vi "Approach_runningAverage_VUW.vi"(7 "Computer called (T/F)":bool) -> ()   [LabVIEW 2023]
uses:
  Sub_Vi/TypeDefsControls/Zposition.ctl
  Sub_Vi/TypeDefsControls/Piezo Velocity.ctl
  Sub_Vi/TypeDefsControls/Voltage.ctl
  Sub_Vi/TypeDefsControls/Xposition.ctl
  Sub_Vi/TypeDefsControls/Yposition.ctl
  Sub_Vi/TypeDefs/WayPointCluster.ctl
  Sub_Vi/TypeDefs/ChangeOnFly.ctl
  Sub_Vi/TypeDefs/Settings.ctl
  Sub_Vi/TypeDefs/Display.ctl
  Sub_Vi/TypeDefsControls/Feedback Type.ctl
  Settings.vi
panel:
  in  "Approach Type":u16=8
  out "Current 1":cluster{"Y":dbl[], "Y":dbl[]}[](graph)
  in  "Boolean Negative":bool
  in  "Boolean Positive":bool=TRUE
  in  "Feedback Type":T1=enum."Current 1"
  in  "Display Cluster":T2
  in  "SettingsCluster":T3={"Sample Rate (us)"=1, "Samples Per Data Point (int, power of 2)"=1000, "DistanceToBulk (um)"=-1.0, "HoldTimeScaler"=1, "SaveData"=TRUE, "DistanceToBulk (um) 2"=-1.0, "DistanceToBulk (um) 3"=-1.0}
  in  "ChangeonFly":T4
  in  "WayPointCluster":T5
  in  "Start scan Button":bool
  in  "Stop":bool
  in  "Pause":bool
  in  "Feedback Threshold (A)\nLower":dbl=-1e-10
  in  "Set X":bool
  in  "Set Y":bool
  in  "Y":T6=100.0 min=0.0 max=100000.0
  in  "X":T7=100.0 min=0.0 max=100000.0
  in  "Approach Voltage (V)":T8 min=-10.0 max=10.0
  in  "Approach Rate (µm/s)":T9=0.1 min=0.0
  in  "End Extension (µm)":T10 min=0.0 max=100000.0
  in  "Start Extention (µm)":T10=150.0 min=0.0 max=100000.0
  out "?":cluster{"Y":dbl[], "Y":dbl[]}[](graph)
  out "?":dbl[](graph)
  # "Settings"
  # "Pause at"
  # "Advanced Settings"
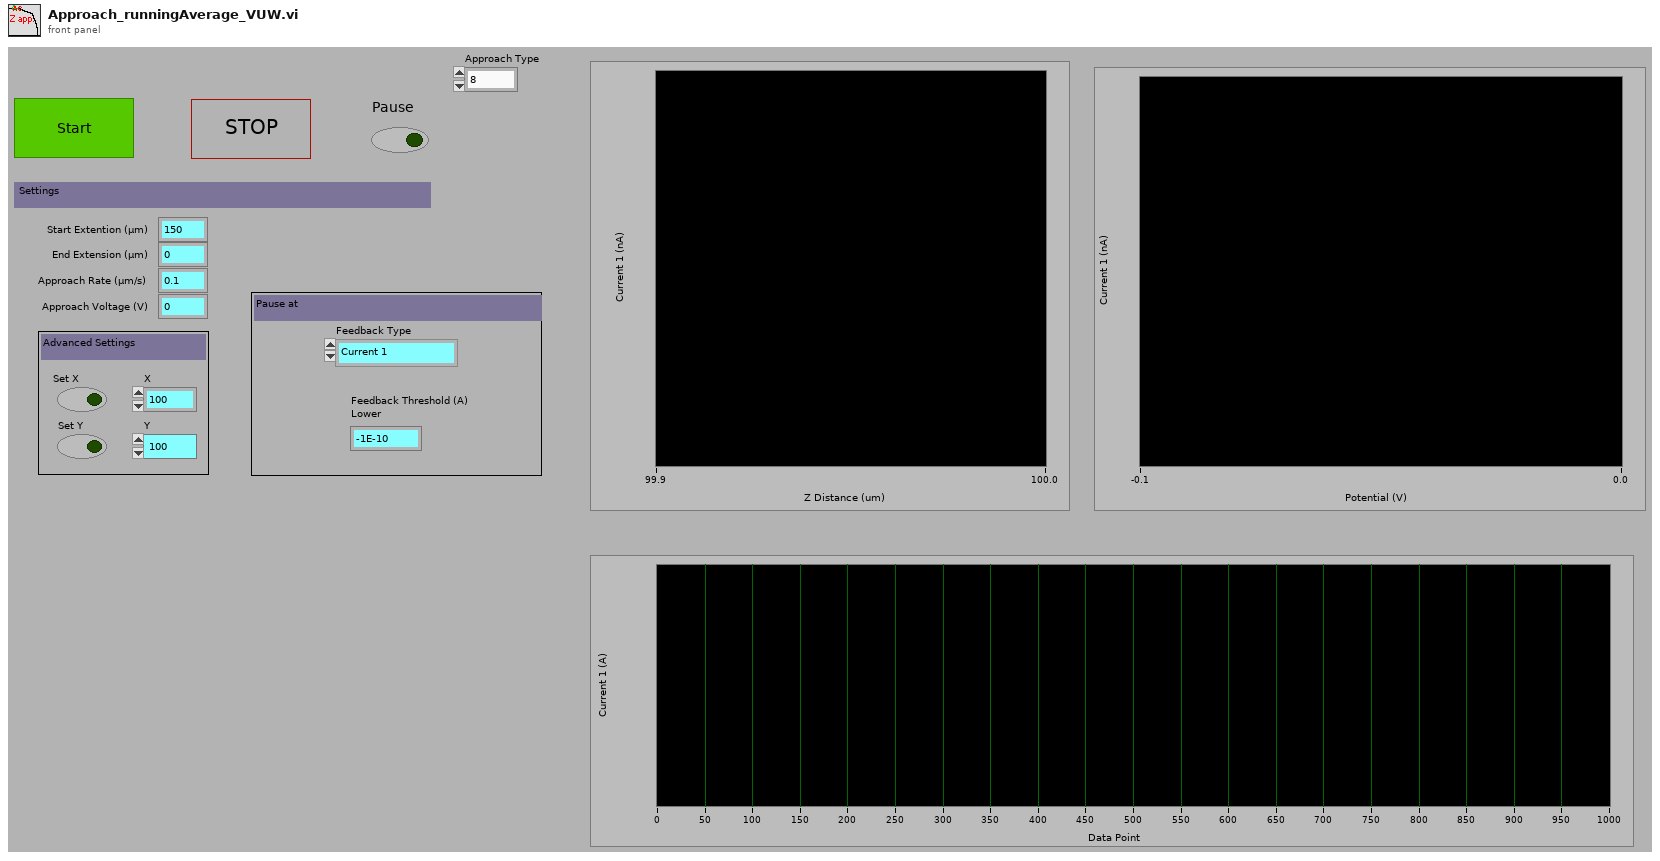
[diagram p1: front panel]
types:
  T1 = typedef "Feedback Type.ctl" = enum16{"AC Magnitude", "Current 1", "Current 2", "Phase"}
  T2 = typedef "Display.ctl" = cluster{"X":refnum<vi>, "Y":refnum<vi>, "Z":refnum<vi>, "Amp":refnum<vi>, "Phase":refnum<vi>, "t vs Z":refnum<vi>, "t vs C1":refnum<vi>, "t vs C2":refnum<vi>, "t vs C3":refnum<vi>, "t vs Amp":refnum<vi>, "t vs Phase":refnum<vi>, "t vs X":refnum<vi>, "t vs Y":refnum<vi>, "Z vs C1":refnum<vi>, "Z vs C2":refnum<vi>, "Z vs C3":refnum<vi>, "V vs C1":refnum<vi>, "V vs C2":refnum<vi>, "V vs C3":refnum<vi>, "X/Y/Z F":refnum<vi>, "X/Y/Z R":refnum<vi>, "X/Y/C1 F":refnum<vi>, "X/Y/C1 R":refnum<vi>, "X/Y/C2 F":refnum<vi>, "X/Y/C2 R":refnum<vi>, "X/Y/C3 F":refnum<vi>, "X/Y/C3 R":refnum<vi>, "NumberOfLines":u16, "um Per Pixel":dbl, "um Per Line":dbl, "X Center":dbl, "Hop X/Y/Z":refnum<vi>, "Hop X/Y/C1":refnum<vi>, "Hop X/Y/C2":refnum<vi>, "Hop X/Y/C3":refnum<vi>, "X Width":dbl, "Y Width":dbl, "Hopping Distance":dbl, "V2 vs C1":refnum<vi>, "V vs Phase":refnum<vi>, "Y Center":dbl, "Number of Pixels":dbl, "V2 vs C2":refnum<vi>, "V2 vs C3":refnum<vi>, "V vs y":refnum<vi>, "V2 vs y":refnum<vi>, "Z vs Amp":refnum<vi>, "Z vs Phase":refnum<vi>}
  T3 = typedef "Settings.ctl" = cluster{"Sample Rate (us)":u32, "Samples Per Data Point (int, power of 2)":i16, "DistanceToBulk (um)":dbl, "HoldTimeScaler":u64, "SaveData":bool, "DistanceToBulk (um) 2":dbl, "DistanceToBulk (um) 3":dbl}
  T4 = typedef "ChangeOnFly.ctl" = cluster{"Stop (boolean)":refnum<vi>, "Pause (boolean)":refnum<vi>, "EndCurrentLine (boolean)":refnum<vi>, "max movement per update step (Interger, nm)":refnum<vi>, "P (float, arb)":refnum<vi>, "Feedback set point (double, Amps)":refnum<vi>, "Voltage (double, V)":refnum<vi>, "Feedback set point 2 (double, Amps)":refnum<vi>, "Stop on Greater Than 2? (boolean)":refnum<vi>, "Stop on Greater Than? (boolean)":refnum<vi>, "Voltage 2 (double, V)":refnum<vi>, "Feedback Type (enum)":refnum<vi>, "Feedback Type 2 (enum)":refnum<vi>}
  T5 = typedef "WayPointCluster.ctl" = cluster{"X (um)":dbl[], "Y (um)":dbl[], "Z (um)":dbl[], "V (V)":dbl[], "X Velocity (um s-1)":dbl[], "Y Velocity (um s-1)":dbl[], "Z Velocity (um s-1)":dbl[], "V Velocity (V s-1)":dbl[], "FeedBack Type (enum)":u16[], "Move X (boolean)":bool[], "Move Y (boolean)":bool[], "Move Z (boolean)":bool[], "Move V (boolean)":bool[], "Jump V (boolean)":bool[], "Hold (boolean)":bool[], "Hold Time":u32[], "V2 (V)":dbl[], "Move V2":bool[], "V2 Velocity (V s-1)":dbl[], "Jump V2 (boolean)":bool[], "Update z Position delta (ms)":i16[], "Hold Feedback1":bool[], "Move Z PicoMotor":bool[], " Z PicoMotor Direction":bool[], "DIO0":bool[]}
  T6 = typedef "Yposition.ctl" = dbl
  T7 = typedef "Xposition.ctl" = dbl
  T8 = typedef "Voltage.ctl" = dbl
  T9 = typedef "Piezo Velocity.ctl" = dbl
  T10 = typedef "Zposition.ctl" = dbl
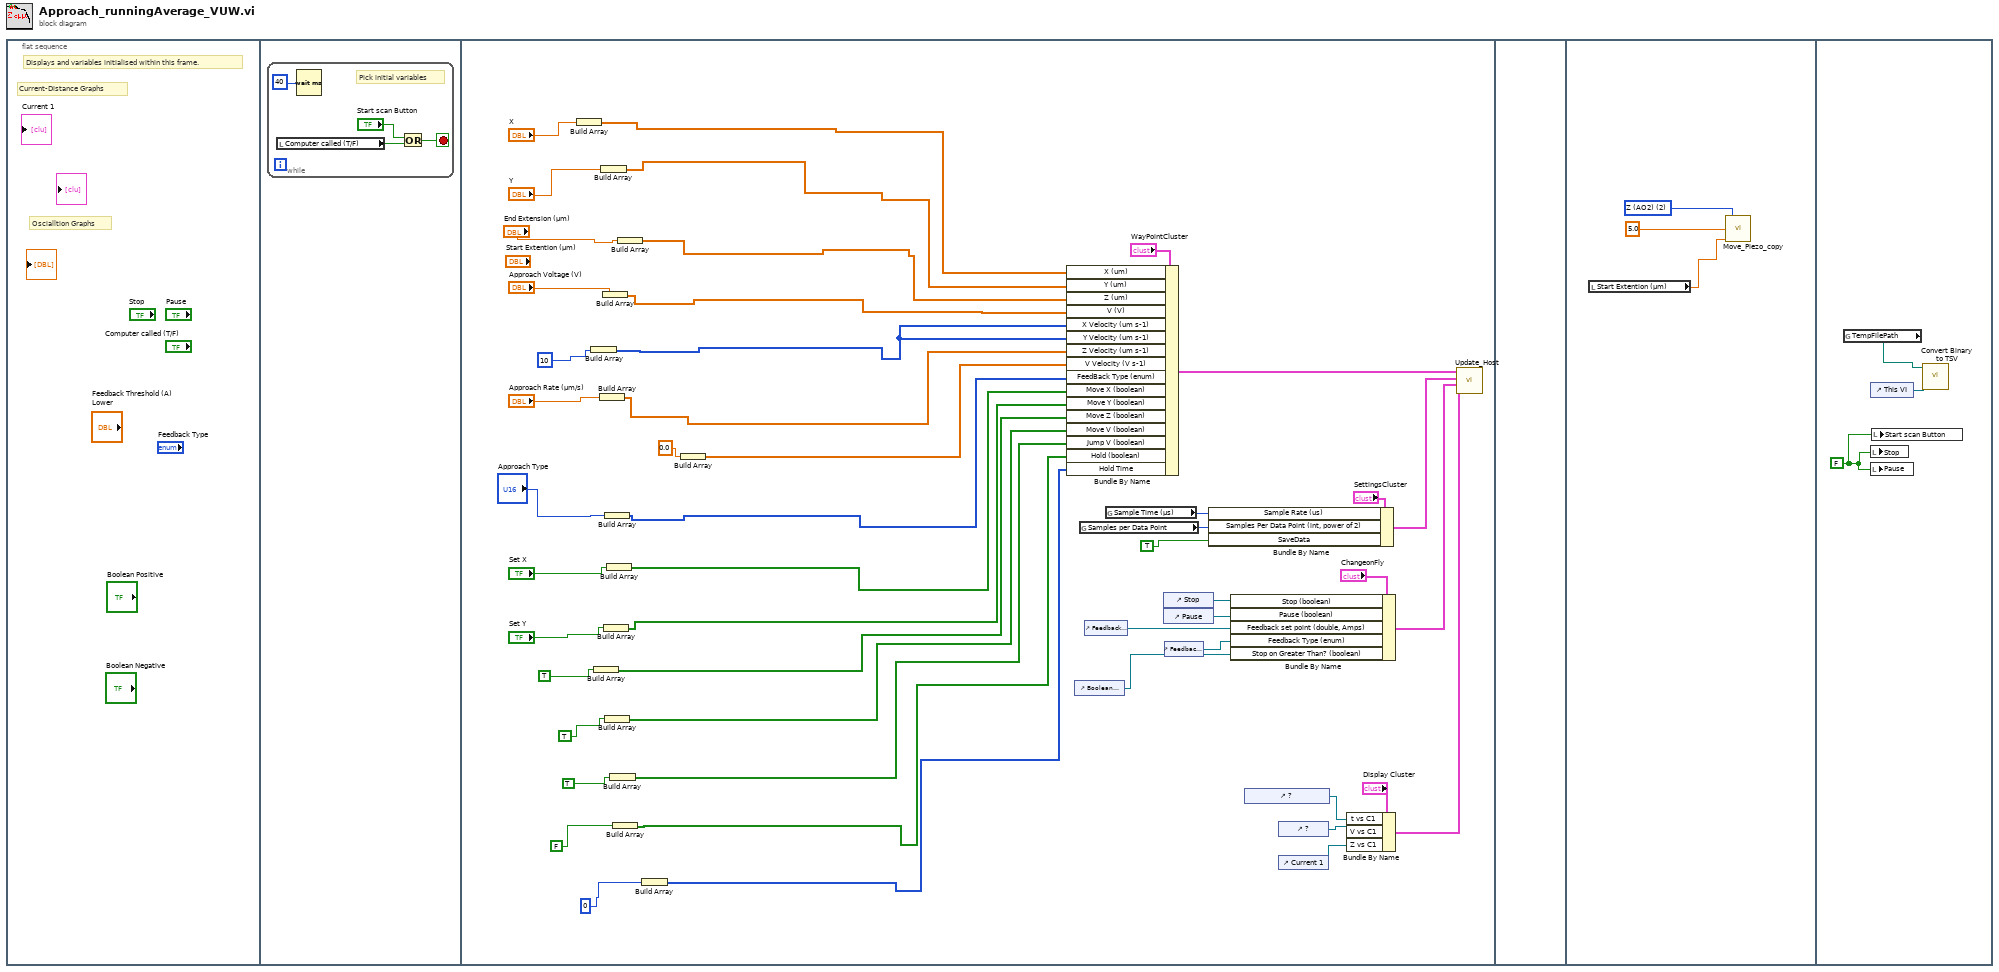
[diagram p0: block diagram]
diagram:
  n1 = flat-sequence {
    frame #0 {
      # "Oscialltion Graphs"
      # "Current-Distance Graphs"
      # "Displays and variables initialised within this frame."
    }
    frame #1 {
      n2 = while {
        stop <- w4 stop-if-true
        # "Pick initial variables"
        n3 = local read "Computer called (T/F)"() -> (w2:bool)
        n4 = Wait (ms)(milliseconds to wait=u32 40) -> ()  [unwired: 1 out]
        n5 = Or(x="Start scan Button", y=w2) -> (x .or. y?=w4:bool)
      }
    }
    frame #2 {
      n6 = Build Array("X") -> (w34:T7[])
      n7 = Build Array(10) -> (w29:i32[])
      n8 = Build Array(TRUE ("Set Z")) -> (w22:bool[])
      n9 = Build Array("Approach Rate (µm/s)") -> (w28:T9[])
      n10 = Build Array("Y") -> (w33:T6[])
      n11 = Build Array("Approach Voltage (V)") -> (w30:T8[])
      n12 = Build Array("Set Y") -> (w23:bool[])
      n13 = Build Array("Approach Type") -> (w26:u16[])
      n14 = Build Array(TRUE ("element")) -> (w21:bool[])
      n15 = Build Array("Set X") -> (w24:bool[])
      n16 = Build Array(TRUE ("Set Z")) -> (w20:bool[])
      n17 = Build Array(FALSE ("Set Z")) -> (w19:bool[])
      n18 = Build Array("End Extension (µm)") -> (w31:T10[])
      n19 = Build Array(u32 0 ("element")) -> (w18:u32[])
      n20 = Build Array(0.0) -> (w27:dbl[])
      n21 = Bundle By Name(cluster="WayPointCluster", "X (um)"=w34, "Y (um)"=w33, "Z (um)"=w31, "V (V)"=w30, "X Velocity (um s-1)"=w29, "Y Velocity (um s-1)"=w29, "Z Velocity (um s-1)"=w28, "V Velocity (V s-1)"=w27, "FeedBack Type (enum)"=w26, "Move X (boolean)"=w24, "Move Y (boolean)"=w23, "Move Z (boolean)"=w22, "Move V (boolean)"=w21, "Jump V (boolean)"=w20, "Hold (boolean)"=w19, "Hold Time"=w18) -> (w53:T5)
      n22 = control-ref of="Boolean Positive"() -> (w36:refnum<vi>)
      n23 = global read "Settings.vi" "Samples per Data Point"() -> (w44:u16)
      n24 = control-ref of="Feedback Threshold (A)\nLower"() -> (w39:refnum<vi>)
      n25 = global read "Settings.vi" "Sample Time (µs)"() -> (w45:u32)
      n26 = control-ref of="Stop"() -> (w49:refnum<vi>)
      n27 = control-ref of="Pause"() -> (w48:refnum<vi>)
      n28 = control-ref of="Feedback Type"() -> (w37:refnum<vi>)
      n29 = Bundle By Name(cluster="SettingsCluster", "Sample Rate (us)"=w45, "Samples Per Data Point (int, power of 2)"=w44, "SaveData"=TRUE) -> (w51:T3)
      n30 = Bundle By Name(cluster="ChangeonFly", "Stop (boolean)"=w49, "Pause (boolean)"=w48, "Feedback set point (double, Amps)"=w39, "Feedback Type (enum)"=w37, "Stop on Greater Than? (boolean)"=w36) -> (w50:T4)
      n31 = control-ref of="?"() -> (w35:refnum<vi>)
      n32 = control-ref of="?"() -> (w43:refnum<vi>)
      n33 = control-ref of="Current 1"() -> (w42:refnum<vi>)
      n34 = Bundle By Name(cluster="Display Cluster", "t vs C1"=w35, "V vs C1"=w43, "Z vs C1"=w42) -> (w52:T2)
      n35 = call "Update_Host.vi"("Display Cluster"=w52, "ChangeonFly"=w50, "SettingsCluster"=w51, "WayPointCluster"=w53) -> ()  [unwired: 6 in]
    }
    frame #3 {
    }
    frame #4 {
      w56 = u16 2 items=["X (AO0)", "Y (AO1)", "Z (AO2)", "V (AO3)", "V2 (AO4)"] ("Piezo")
      n36 = local read "Start Extention (µm)"() -> (w54:T10)
      n37 = call "Move_Piezo_copy.vi"("Piezo"=w56, "Movement Speed (µm/s)"=5.0 ("Scan Rate (um/s)"), "Position (µm) (or V)"=w54) -> ()  [unwired: 13 in]
    }
    frame #5 {
      w58 = FALSE ("Start Scanning Button")
      n38 = global read "Settings.vi" "TempFilePath"() -> (w57:path)
      n39 = control-ref of="This VI"() -> (w59:refnum<vi>)
      n40 = local write "Stop"(w58) -> ()
      n41 = local write "Pause"(w58) -> ()
      n42 = local write "Start scan Button"(w58) -> ()
      n43 = call "Convert Binary to TSV.vi"("This VI"=w59, "TDMS DataFile Name"=w57) -> ()  [unwired: 10 in]
    }
  }
